vi "get_JSON_string.vi"(3 "error in (no error)":errorcluster, 4 "field name":string, 5 "metadata JSON string":string) -> (0 "error out":errorcluster, 2 "JSON string":string)   [LabVIEW 2011, in "Rinocloud Library.lvlib"]
uses:
  Rinocloud Library.lvlib
  i3 JSON/i3-json.lvlib
  i3 JSON/JSON Parsing/Get Object Parameter Files/Get Object Parameter - Array.vi
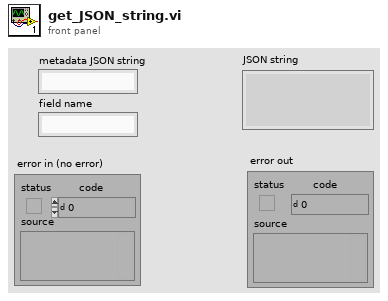
[diagram p1: front panel]
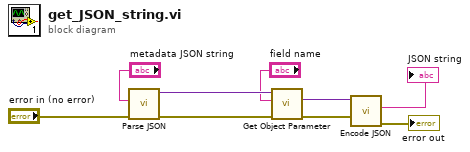
[diagram p0: block diagram]
diagram:
  n1 = call "Parse JSON.vi"("error in (no error)"="error in (no error)", "JSON String"="metadata JSON string") -> ("error out"=w7:errorcluster, "JSON Tree"=w8:variant)  [unwired: 6 in, 2 out]
  n2 = call-poly "Get Object Parameter.vi"("error in (no error)"=w7, "Parameter Name"="field name", "JSON Tree In (JSON Object)"=w8) -> ("error out"=w3:errorcluster, "JSON Array"=w4:variant)  [unwired: 5 in, 2 out]
  n3 = call "Encode JSON.vi"("error in (no error)"=w3, "JSON Tree"=w4) -> ("error out"=→"error out":errorcluster, "String"=→"JSON string":string)  [unwired: 4 in]
